vi "GM Count 12-09-06.vi"() -> ()   [LabVIEW 2010]
uses:
  <vilib>/DAQmx/read.llb/DAQmx Read (Counter U32 1Chan 1Samp).vi
  <vilib>/DAQmx/create/channels.llb/DAQmx Create Channel (CI-Count Edges).vi
  <vilib>/daqmx/miscellaneous.llb/DAQmx Fill In Error Info.vi
  <vilib>/DAQmx/configure/timing.llb/DAQmx Timing (Sample Clock).vi
panel:
  in  "stop":bool
  in  "Seconds to Count":dbl=1.0
  out "Counts":u32
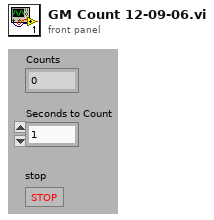
[diagram p1: front panel]
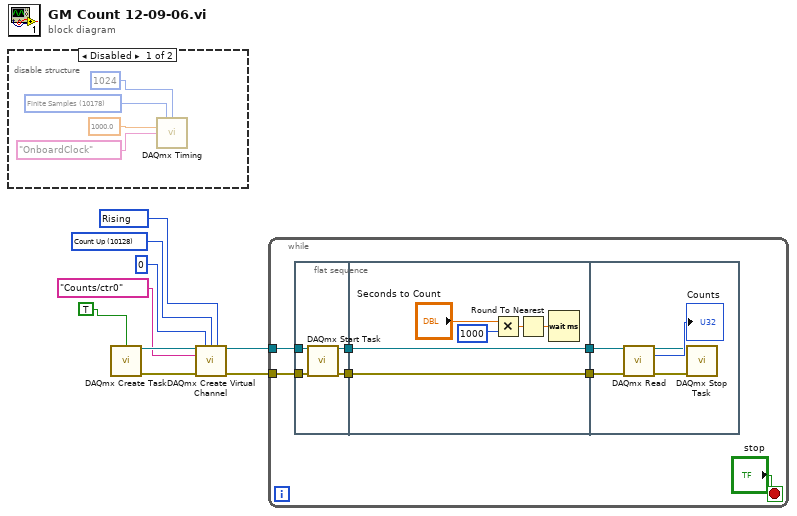
[diagram p0: block diagram]
diagram:
  w3 = 10280 items=["Rising"=10280, "Falling"=10171] ("edge")
  w4 = 10128 items=["Count Up"=10128, "Count Down"=10124, "Externally Controlled"=10326] ("count direction")
  n1 = disable-structure shown="Disabled" {
    frame Disabled {
      w13 = 10178 items=["Finite Samples"=10178, "Continuous Samples"=10123, "Hardware Timed Single Point"=12522] ("sample mode")
      n2 = call-poly <vilib>:"DAQmx Timing.vi"("sample mode"=w13, "samples per channel"=1024, "rate"=1000.0, "source"=tag "OnboardClock") -> ()  [unwired: 10 in, 2 out]
    }
    frame Enabled {
    }
  }
  n3 = call <vilib>:"DAQmx Create Task.vi"("auto cleanup"=TRUE) -> ("task out"=w8:refnum<k21>, "error out"=w7:errorcluster)  [unwired: 13 in]
  n4 = call-poly <vilib>:"DAQmx Create Virtual Channel.vi"("task in"=w8, "initial count"=u32 0, "count direction"=w4, "edge"=w3, "counter"=tag "Counts/ctr0", "error in"=w7) -> ("task out"=w1:refnum<k21>, "error out"=w2:errorcluster)  [unwired: 8 in]
  n5 = while {
    tunnel: w2 -> [w20]
    tunnel: w1 -> [w19]
    stop <- "stop" stop-if-true
    n6 = flat-sequence {
      tunnel: w20 -> [w24]
      tunnel: w19 -> [w23]
      tunnel: [w22] -> w18
      tunnel: [w21] -> w17
      tunnel: w18 -> [w30]
      tunnel: w17 -> [w29]
      tunnel: [w30] -> w16
      tunnel: [w29] -> w15
      tunnel: w16 -> [w31]
      tunnel: w15 -> [w32]
      frame #0 {
        n7 = call <vilib>:"DAQmx Start Task.vi"("task/channels in"=w23, "error in"=w24) -> ("task out"=w22:refnum<k21>, "error out"=w21:errorcluster)  [unwired: 12 in]
      }
      frame #1 {
        n8 = Multiply(x="Seconds to Count", y=u32 1000) -> (x*y=w26:dbl)
        n9 = Round To Nearest(number=w26) -> (nearest integer value=w25:dbl)
        n10 = Wait (ms)(milliseconds to wait=w25) -> ()  [unwired: 1 out]
      }
      frame #2 {
        n11 = call-poly <vilib>:"DAQmx Read.vi"("task/channels in"=w31, "error in"=w32) -> ("task out"=w34:refnum<k21>, "data"=→"Counts":u32, "error out"=w33:errorcluster)  [unwired: 11 in]
        n12 = call <vilib>:"DAQmx Stop Task.vi"("task/channels in"=w34, "error in"=w33) -> ()  [unwired: 12 in, 2 out]
      }
    }
  }
